vi "FoolishDriver.vi"(1 "AutoEnable":bool, 2 "AutoMode":T2) -> ()   [LabVIEW 2019]
uses:
  TypeDefs/AutoMode.ctl
  ArgosLib/Signal Processing/TypeDefs/EdgeDetector_Type.ctl
  Global_Var-RefNum/RobotState.vi
  Global_Var-RefNum/AutoCommands.vi
  ArgosLib/ArgosLib.lvlib
panel:
  out "RoutineStage":i32
  in  "Tab Control":T1(tab)=enum."FriendlyTrench"
  in  "MaxRampRate(%/s)":dbl=0.5
  in  "MaxSpeed":dbl=0.5
  in  "Distance(in)":dbl=36.0
  in  "ShootTime(ms)":u32=3000
  in  "ShootThenDrivePrimeSpeed":dbl=3000.0
  in  "MaxRampRate(%/s) 2":dbl=0.5
  in  "MaxSpeed 2":dbl=0.5
  in  "Distance(in) 2":dbl=36.0
  in  "ShootThenDrivePrimeSpeed 2":dbl=3000.0
  in  "ShootTime(ms) 2":u32=3000
  in  "Distance(in) 3":dbl=36.0
  in  "MaxSpeed 3":dbl=0.5
  in  "MaxRampRate(%/s) 3":dbl=0.5
  in  "ShootThenDrivePrimeSpeed 3":dbl=3000.0
  in  "ShootTime(ms) 3":u32=3000
  in  "Distance(in) 4":dbl=72.0
  in  "MaxSpeed 4":dbl=0.75
  in  "MaxRampRate(%/s) 4":dbl=0.5
  in  "Distance(in) 5":dbl=-72.0
  in  "MaxSpeed 5":dbl=0.75
  in  "MaxRampRate(%/s) 5":dbl=0.5
  in  "ShootThenDrivePrimeSpeed 4":dbl=3000.0
  in  "ShootTime(ms) 4":u32=3000
  in  "Distance(in) 6":dbl=120.0
  in  "MaxSpeed 6":dbl=0.75
  in  "MaxRampRate(%/s) 6":dbl=0.5
  in  "ShootTime(ms) 5":u32=3000
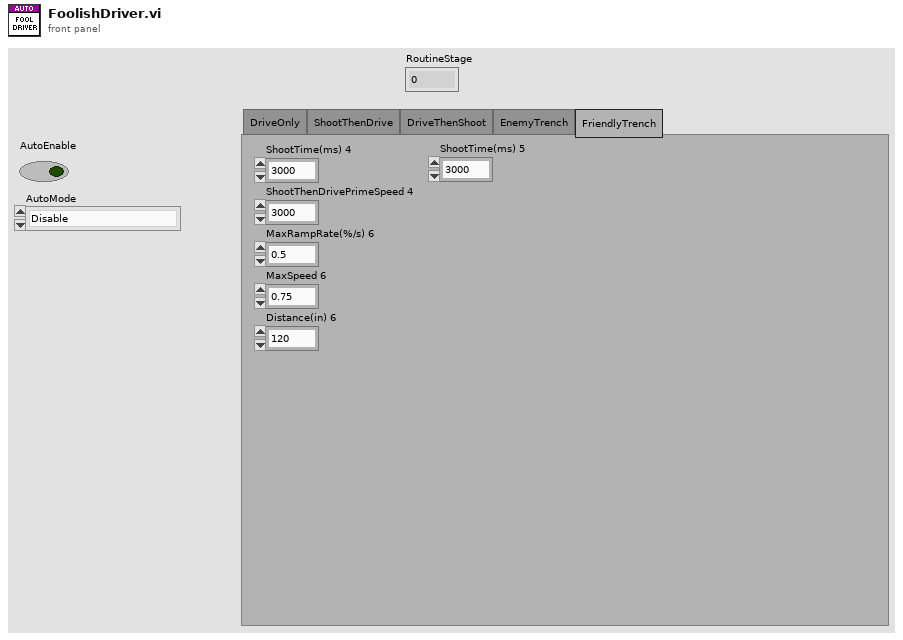
[diagram p1: front panel]
types:
  T1 = enum32{"DriveOnly", "ShootThenDrive", "DriveThenShoot", "EnemyTrench", "FriendlyTrench"}
  T2 = typedef "AutoMode.ctl" = enum16{"Disable", "DriveOnly", "ShootThenDrive", "DriveThenShoot", "EnemyTrench", "FriendlyTrench"}
  T3 = typedef "ArgosLib.lvlib/EdgeDetector_Type.ctl" = enum16{"RisingEdge", "FallingEdge", "Both"}
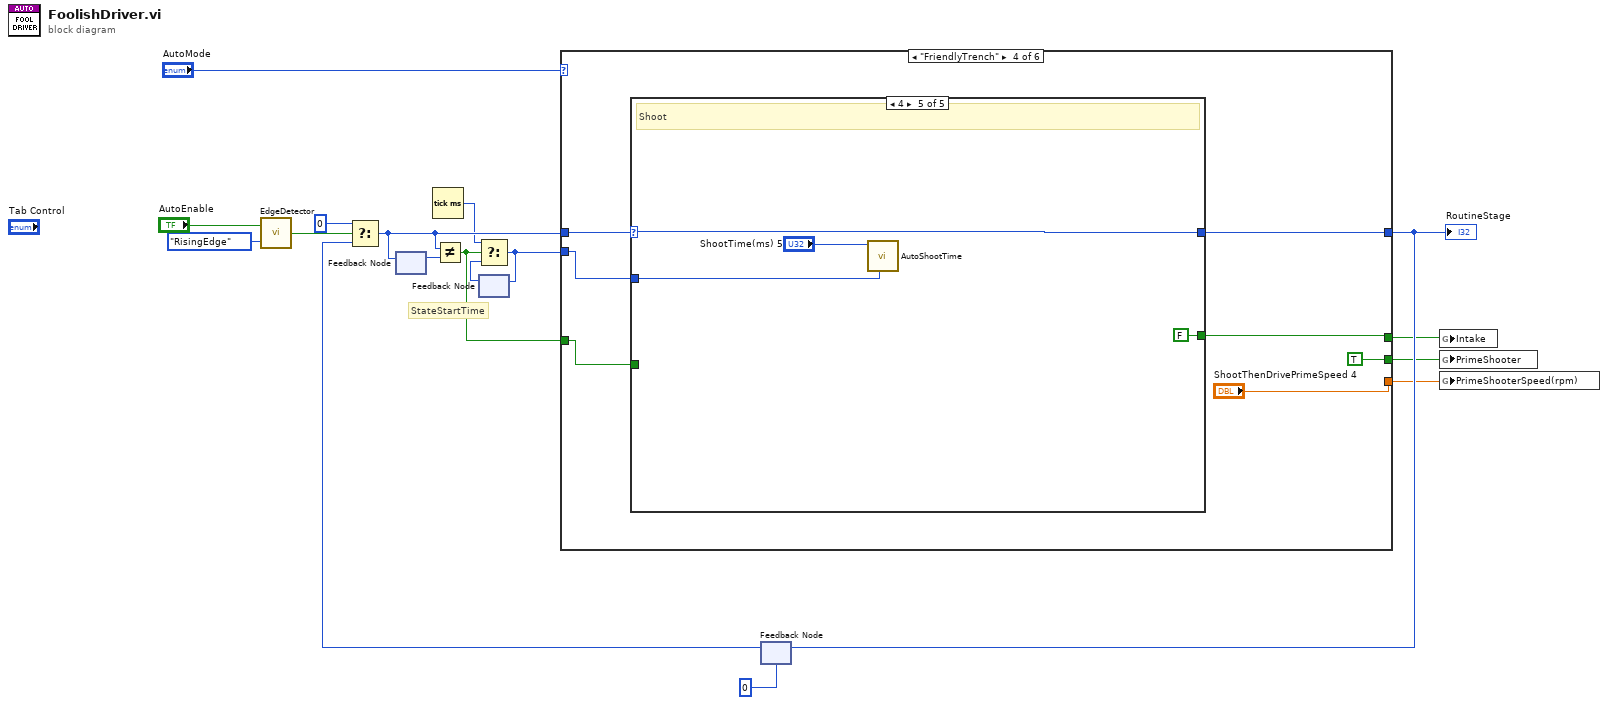
[diagram p0: block diagram]
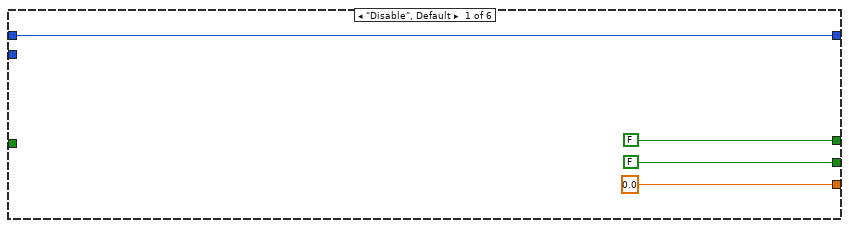
[diagram p2: hidden frame]
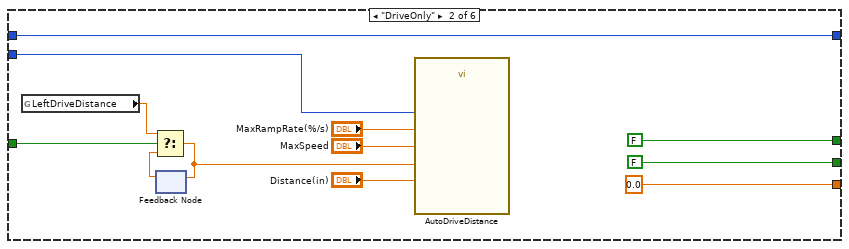
[diagram p3: hidden frame]
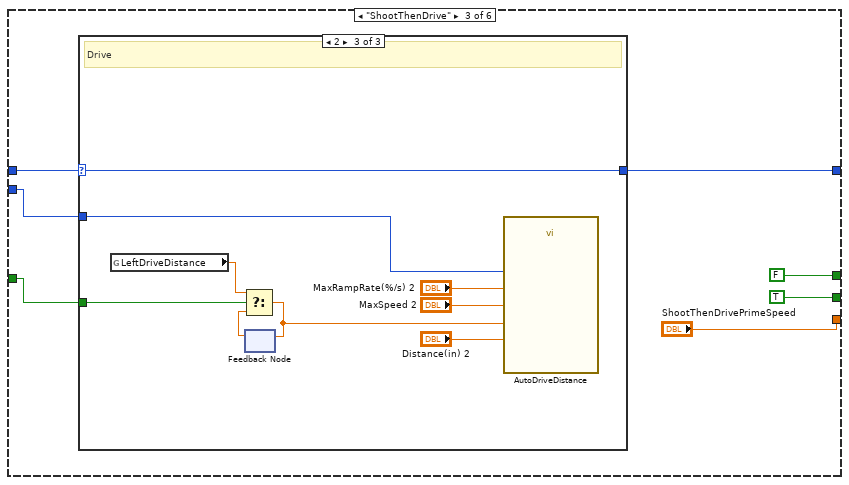
[diagram p4: hidden frame]
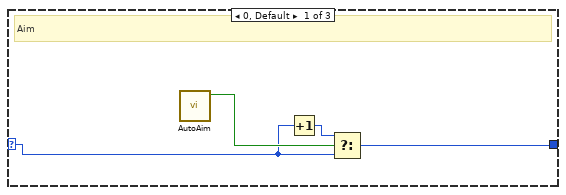
[diagram p5: hidden frame]
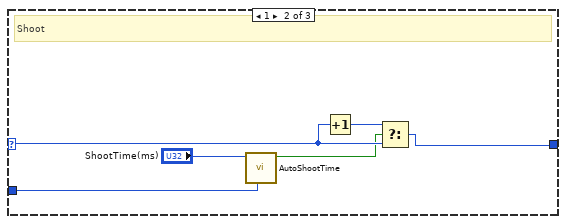
[diagram p6: hidden frame]
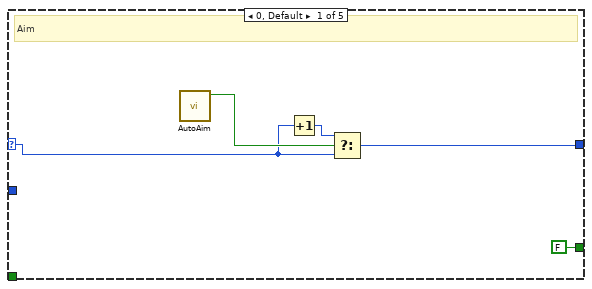
[diagram p7: hidden frame]
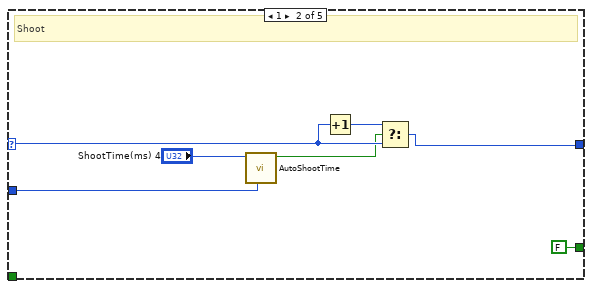
[diagram p8: hidden frame]
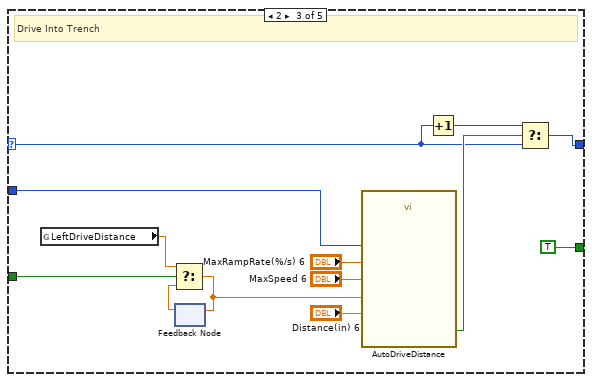
[diagram p9: hidden frame]
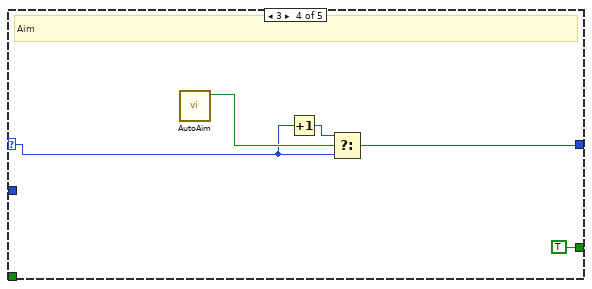
[diagram p10: hidden frame]
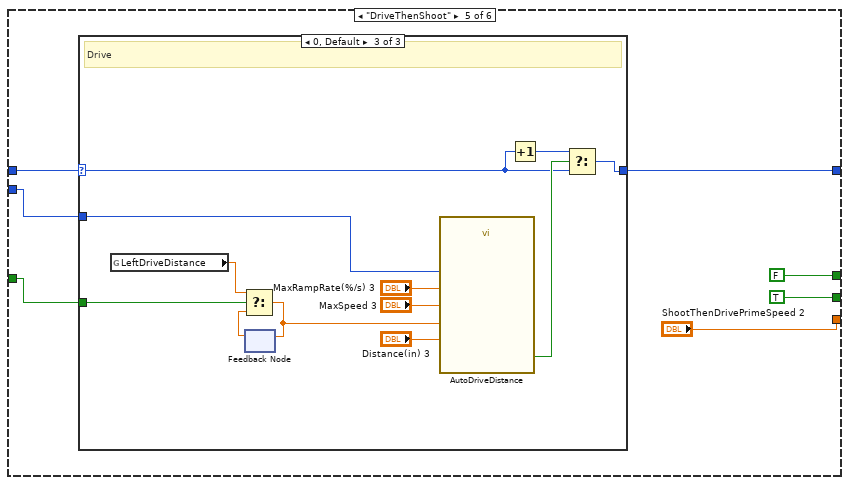
[diagram p11: hidden frame]
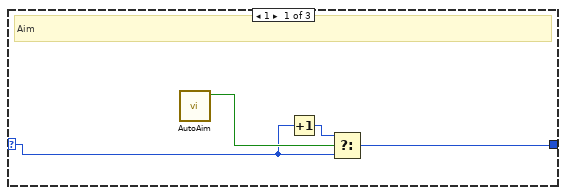
[diagram p12: hidden frame]
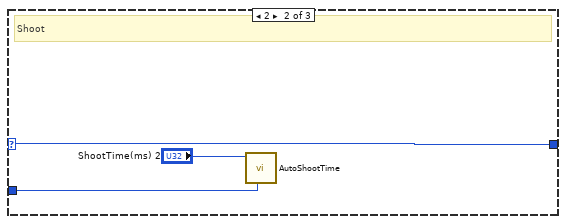
[diagram p13: hidden frame]
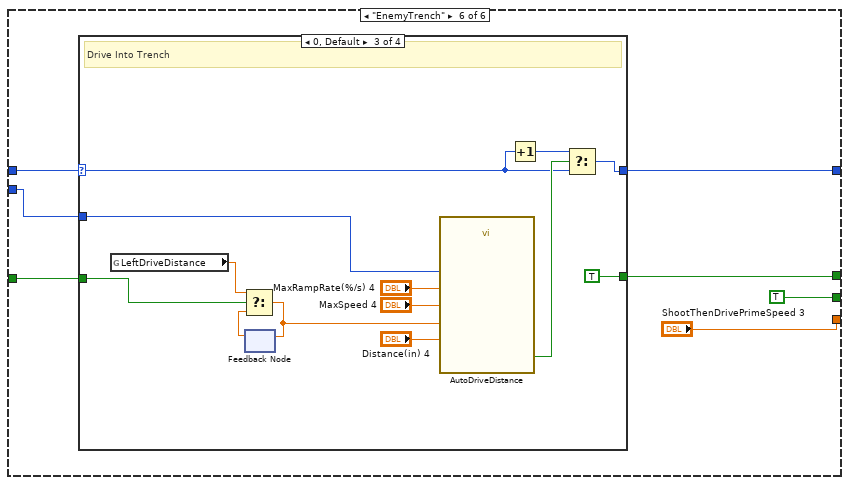
[diagram p14: hidden frame]
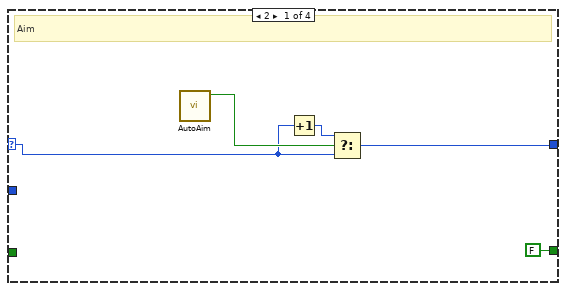
[diagram p15: hidden frame]
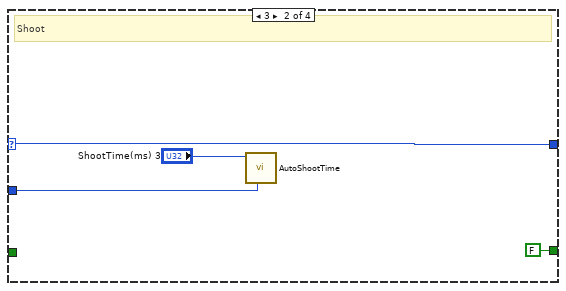
[diagram p16: hidden frame]
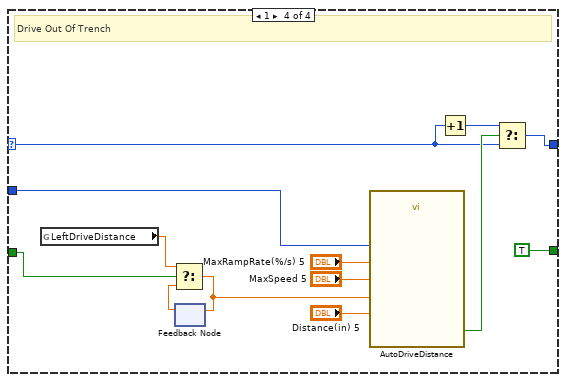
[diagram p17: hidden frame]
diagram:
  # "StateStartTime"
  n1 = call "EdgeDetector.vi"("DetectorType"=EdgeDetector_Type."RisingEdge", "Input"="AutoEnable") -> ("Edge"=w13:bool)
  n2 = feedback #1() -> (w9:i32)  [unwired: 1 in]
  n3 = Tick Count (ms)() -> (millisecond timer value=w7:u32)
  n4 = feedback #2() -> (w6:u32)  [unwired: 1 in]
  n5 = feedback #3(0) -> (w12:i32)
  n6 = Select(t=0, s=w13, f=w12) -> (s? t:f=w8:i32)
  n7 = feedback-in #1(w8) -> ()
  n8 = Not Equal?(x=w8, y=w9) -> (x != y?=w4:bool)
  n9 = Select(t=w7, s=w4, f=w6) -> (s? t:f=w5:u32)
  n10 = feedback-in #2(w5) -> ()
  n11 = case shown="\"FriendlyTrench\"" "AutoMode" {
    tunnel: w8 -> [w21 w32 w40 w66 w107 w133]
    tunnel: [w21 w32 w39 w65 w106 w132] -> w10
    tunnel: w5 -> [_ w33 w38 w64 w105 w131]
    tunnel: w4 -> [_ w28 w34 w61 w101 w127]
    tunnel: [FALSE ("Intake") FALSE ("Intake") FALSE ("Intake") w60 FALSE ("Intake") w128] -> w3
    tunnel: [FALSE ("PrimeShooter") FALSE ("PrimeShooter") TRUE ("PrimeShooter") TRUE ("PrimeShooter") TRUE ("PrimeShooter") TRUE ("PrimeShooter")] -> w2
    tunnel: [0.0 ("PrimeShooterSpeed(rpm)") 0.0 ("PrimeShooterSpeed(rpm)") "ShootThenDrivePrimeSpeed" "ShootThenDrivePrimeSpeed 4" "ShootThenDrivePrimeSpeed 2" "ShootThenDrivePrimeSpeed 3"] -> w1
    frame "Disable", Default {
    }
    frame "DriveOnly" {
      n12 = global read "RobotState.vi" "LeftDriveDistance"() -> (w27:dbl)
      n13 = feedback #4() -> (w26:dbl)  [unwired: 1 in]
      n14 = Select(t=w27, s=w28, f=w26) -> (s? t:f=w25:dbl)
      n15 = feedback-in #4(w25) -> ()
      n16 = call "AutoDriveDistance.vi"("StartTime(ms)"=w33, "MaxRampRate(%/s)"="MaxRampRate(%/s)", "MaxSpeed"="MaxSpeed", "Distance(in)"="Distance(in)", "StartDistance"=w25) -> ()  [unwired: 6 in, 1 out]
    }
    frame "ShootThenDrive" {
      n17 = case shown="2" w40 {
        selector: w40 -> [w41 w47 w52]
        tunnel: [w43 w48 w52] -> w39
        tunnel: w38 -> [_ w50 w53]
        tunnel: w34 -> [_ _ w51]
        frame 0, Default {
          # "Aim"
          n18 = call "AutoAim.vi"() -> ("Complete"=w44:bool)  [unwired: 11 in]
          n19 = Increment(x=w41) -> (x+1=w42:i32)
          n20 = Select(t=w42, s=w44, f=w41) -> (s? t:f=w43:i32)
        }
        frame 1 {
          # "Shoot"
          n21 = call "AutoShootTime.vi"("StartTime(ms)"=w50, "ShootTime(ms)"="ShootTime(ms)") -> ("Complete"=w45:bool)  [unwired: 9 in]
          n22 = Increment(x=w47) -> (x+1=w46:i32)
          n23 = Select(t=w46, s=w45, f=w47) -> (s? t:f=w48:i32)
        }
        frame 2 {
          # "Drive"
          n24 = global read "RobotState.vi" "LeftDriveDistance"() -> (w56:dbl)
          n25 = feedback #5() -> (w55:dbl)  [unwired: 1 in]
          n26 = Select(t=w56, s=w51, f=w55) -> (s? t:f=w54:dbl)
          n27 = feedback-in #5(w54) -> ()
          n28 = call "AutoDriveDistance.vi"("StartTime(ms)"=w53, "MaxRampRate(%/s)"="MaxRampRate(%/s) 2", "MaxSpeed"="MaxSpeed 2", "Distance(in)"="Distance(in) 2", "StartDistance"=w54) -> ()  [unwired: 6 in, 1 out]
        }
      }
    }
    frame "FriendlyTrench" {
      n29 = case shown="4" w66 {
        selector: w66 -> [w68 w75 w80 w93 w97]
        tunnel: [w70 w76 w79 w95 w97] -> w65
        tunnel: w64 -> [_ w78 w85 _ w100]
        tunnel: w61 -> [_ _ w84 _ _]
        tunnel: [FALSE ("Intake") FALSE ("Intake") TRUE ("Intake") TRUE ("Intake") FALSE ("Intake")] -> w60
        frame 0, Default {
          # "Aim"
          n30 = call "AutoAim.vi"() -> ("Complete"=w71:bool)  [unwired: 11 in]
          n31 = Increment(x=w68) -> (x+1=w69:i32)
          n32 = Select(t=w69, s=w71, f=w68) -> (s? t:f=w70:i32)
        }
        frame 1 {
          # "Shoot"
          n33 = call "AutoShootTime.vi"("StartTime(ms)"=w78, "ShootTime(ms)"="ShootTime(ms) 4") -> ("Complete"=w73:bool)  [unwired: 9 in]
          n34 = Increment(x=w75) -> (x+1=w74:i32)
          n35 = Select(t=w74, s=w73, f=w75) -> (s? t:f=w76:i32)
        }
        frame 2 {
          # "Drive Into Trench"
          n36 = global read "RobotState.vi" "LeftDriveDistance"() -> (w88:dbl)
          n37 = feedback #6() -> (w87:dbl)  [unwired: 1 in]
          n38 = Select(t=w88, s=w84, f=w87) -> (s? t:f=w86:dbl)
          n39 = feedback-in #6(w86) -> ()
          n40 = call "AutoDriveDistance.vi"("StartTime(ms)"=w85, "MaxRampRate(%/s)"="MaxRampRate(%/s) 6", "MaxSpeed"="MaxSpeed 6", "Distance(in)"="Distance(in) 6", "StartDistance"=w86) -> ("Complete"=w82:bool)  [unwired: 6 in]
          n41 = Increment(x=w80) -> (x+1=w81:i32)
          n42 = Select(t=w81, s=w82, f=w80) -> (s? t:f=w79:i32)
        }
        frame 3 {
          # "Aim"
          n43 = call "AutoAim.vi"() -> ("Complete"=w96:bool)  [unwired: 11 in]
          n44 = Increment(x=w93) -> (x+1=w94:i32)
          n45 = Select(t=w94, s=w96, f=w93) -> (s? t:f=w95:i32)
        }
        frame 4 {
          # "Shoot"
          n46 = call "AutoShootTime.vi"("StartTime(ms)"=w100, "ShootTime(ms)"="ShootTime(ms) 5") -> ()  [unwired: 9 in, 1 out]
        }
      }
    }
    frame "DriveThenShoot" {
      n47 = case shown="0, Default" w107 {
        selector: w107 -> [w108 w112 w116]
        tunnel: [w110 w112 w118] -> w106
        tunnel: w105 -> [_ w114 w120]
        tunnel: w101 -> [_ _ w115]
        frame 1 {
          # "Aim"
          n48 = call "AutoAim.vi"() -> ("Complete"=w111:bool)  [unwired: 11 in]
          n49 = Increment(x=w108) -> (x+1=w109:i32)
          n50 = Select(t=w109, s=w111, f=w108) -> (s? t:f=w110:i32)
        }
        frame 2 {
          # "Shoot"
          n51 = call "AutoShootTime.vi"("StartTime(ms)"=w114, "ShootTime(ms)"="ShootTime(ms) 2") -> ()  [unwired: 9 in, 1 out]
        }
        frame 0, Default {
          # "Drive"
          n52 = global read "RobotState.vi" "LeftDriveDistance"() -> (w123:dbl)
          n53 = feedback #7() -> (w122:dbl)  [unwired: 1 in]
          n54 = Select(t=w123, s=w115, f=w122) -> (s? t:f=w121:dbl)
          n55 = feedback-in #7(w121) -> ()
          n56 = call "AutoDriveDistance.vi"("StartTime(ms)"=w120, "MaxRampRate(%/s)"="MaxRampRate(%/s) 3", "MaxSpeed"="MaxSpeed 3", "Distance(in)"="Distance(in) 3", "StartDistance"=w121) -> ("Complete"=w119:bool)  [unwired: 6 in]
          n57 = Increment(x=w116) -> (x+1=w117:i32)
          n58 = Select(t=w117, s=w119, f=w116) -> (s? t:f=w118:i32)
        }
      }
    }
    frame "EnemyTrench" {
      n59 = case shown="0, Default" w133 {
        selector: w133 -> [w135 w140 w145 w158]
        tunnel: [w137 w140 w147 w160] -> w132
        tunnel: w131 -> [_ w142 w149 w162]
        tunnel: [FALSE ("Intake") FALSE ("Intake") TRUE ("Intake") TRUE ("Intake")] -> w128
        tunnel: w127 -> [_ _ w143 w156]
        frame 2 {
          # "Aim"
          n60 = call "AutoAim.vi"() -> ("Complete"=w138:bool)  [unwired: 11 in]
          n61 = Increment(x=w135) -> (x+1=w136:i32)
          n62 = Select(t=w136, s=w138, f=w135) -> (s? t:f=w137:i32)
        }
        frame 3 {
          # "Shoot"
          n63 = call "AutoShootTime.vi"("StartTime(ms)"=w142, "ShootTime(ms)"="ShootTime(ms) 3") -> ()  [unwired: 9 in, 1 out]
        }
        frame 0, Default {
          # "Drive Into Trench"
          n64 = global read "RobotState.vi" "LeftDriveDistance"() -> (w152:dbl)
          n65 = feedback #8() -> (w151:dbl)  [unwired: 1 in]
          n66 = Select(t=w152, s=w143, f=w151) -> (s? t:f=w150:dbl)
          n67 = feedback-in #8(w150) -> ()
          n68 = call "AutoDriveDistance.vi"("StartTime(ms)"=w149, "MaxRampRate(%/s)"="MaxRampRate(%/s) 4", "MaxSpeed"="MaxSpeed 4", "Distance(in)"="Distance(in) 4", "StartDistance"=w150) -> ("Complete"=w148:bool)  [unwired: 6 in]
          n69 = Increment(x=w145) -> (x+1=w146:i32)
          n70 = Select(t=w146, s=w148, f=w145) -> (s? t:f=w147:i32)
        }
        frame 1 {
          # "Drive Out Of Trench"
          n71 = global read "RobotState.vi" "LeftDriveDistance"() -> (w165:dbl)
          n72 = feedback #9() -> (w164:dbl)  [unwired: 1 in]
          n73 = Select(t=w165, s=w156, f=w164) -> (s? t:f=w163:dbl)
          n74 = feedback-in #9(w163) -> ()
          n75 = call "AutoDriveDistance.vi"("StartTime(ms)"=w162, "MaxRampRate(%/s)"="MaxRampRate(%/s) 5", "MaxSpeed"="MaxSpeed 5", "Distance(in)"="Distance(in) 5", "StartDistance"=w163) -> ("Complete"=w161:bool)  [unwired: 6 in]
          n76 = Increment(x=w158) -> (x+1=w159:i32)
          n77 = Select(t=w159, s=w161, f=w158) -> (s? t:f=w160:i32)
        }
      }
    }
  }
  "RoutineStage" <- w10
  n78 = feedback-in #3(w10) -> ()
  n79 = global write "AutoCommands.vi" "Intake"(w3) -> ()
  n80 = global write "AutoCommands.vi" "PrimeShooter"(w2) -> ()
  n81 = global write "AutoCommands.vi" "PrimeShooterSpeed(rpm)"(w1) -> ()
